vi "数据查询_仪器日志.vi"() -> ()   [LabVIEW 2016]
uses:
  <vilib>/Utility/miscctls.llb/LVRowAndColumnUnsignedTypeDef.ctl
  <vilib>/Utility/miscctls.llb/LVPointTypeDef.ctl
  <userlib>/_OpenG.lib/array/array.llb/Sort 2D Array (String)__ogtk.vi
panel:
  in  "序列号":string
  out "总共行数":i32
  in  "显示行数":i32=15
  in  "下拉列表":string(xcontrol)
  in  "导出":bool
  in  "查询":bool
  out "数据表":string[][](table)
  in  "结束日期":string="2050/01/01"
  in  "起始日期":string="2010/01/01"
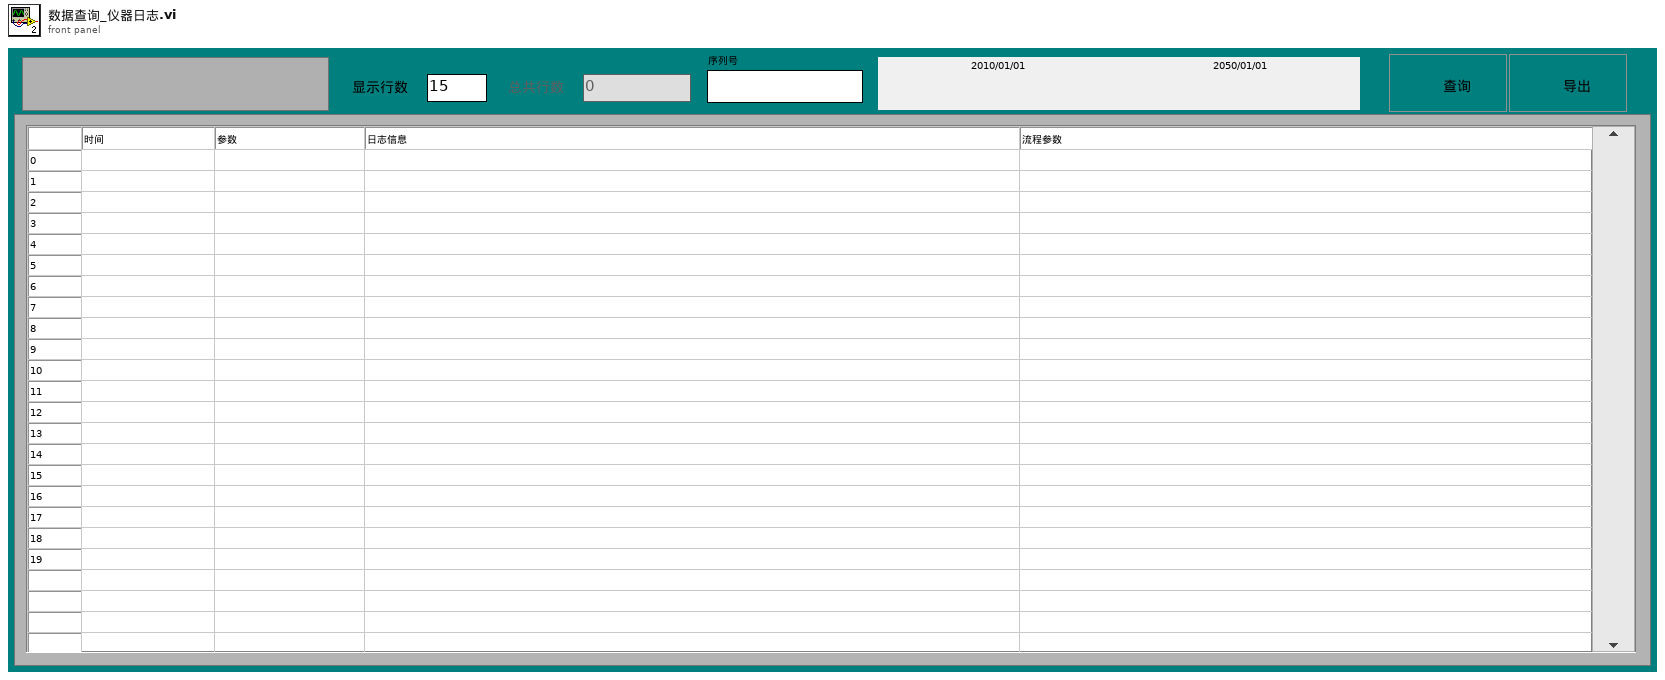
[diagram p1: front panel]
types:
  T1 = enum8{"Enabled", "Disabled", "Disabled and Grayed Out"}
  T2 = typedef "LVRowAndColumnUnsignedTypeDef.ctl" = cluster{"Row":u32, "Column":u32}
  T3 = typedef "LVPointTypeDef.ctl" = cluster{"Horizontal":i16, "Vertical":i16}
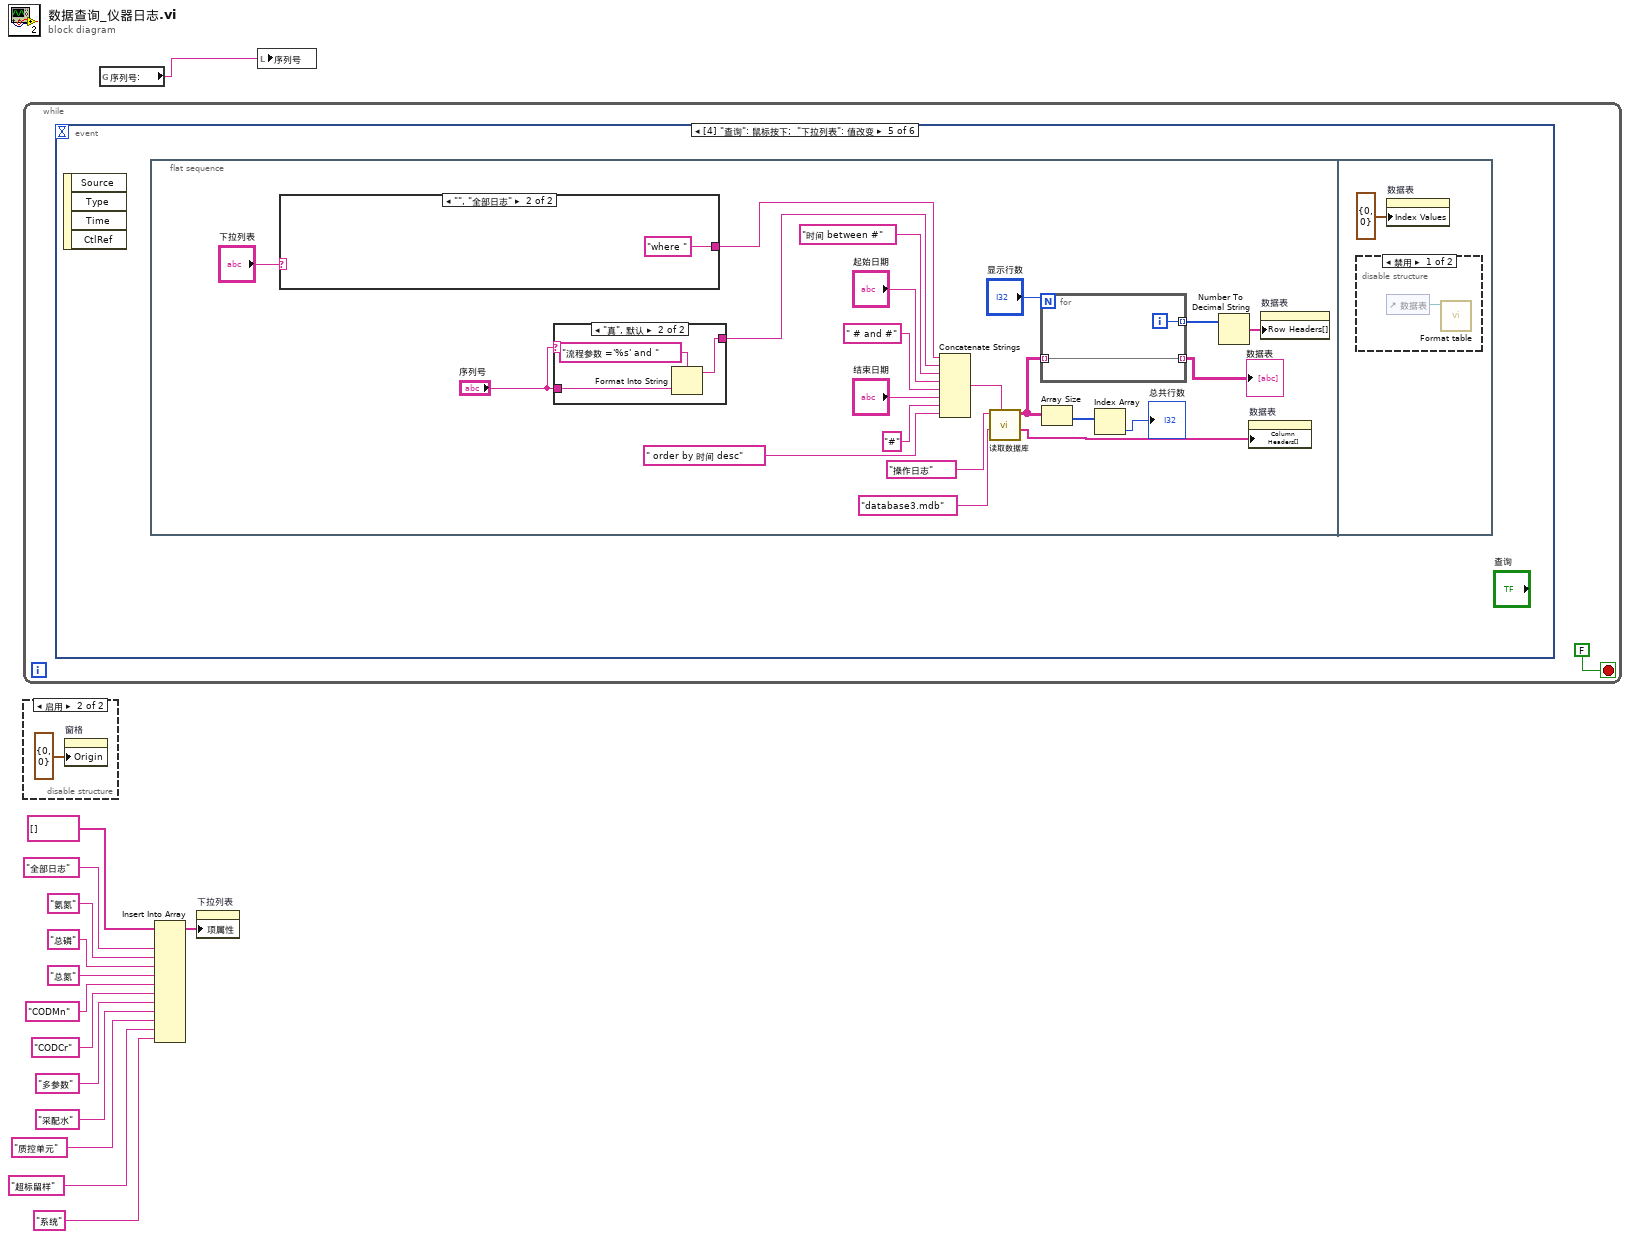
[diagram p0: block diagram]
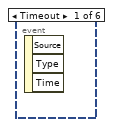
[diagram p2: hidden frame]
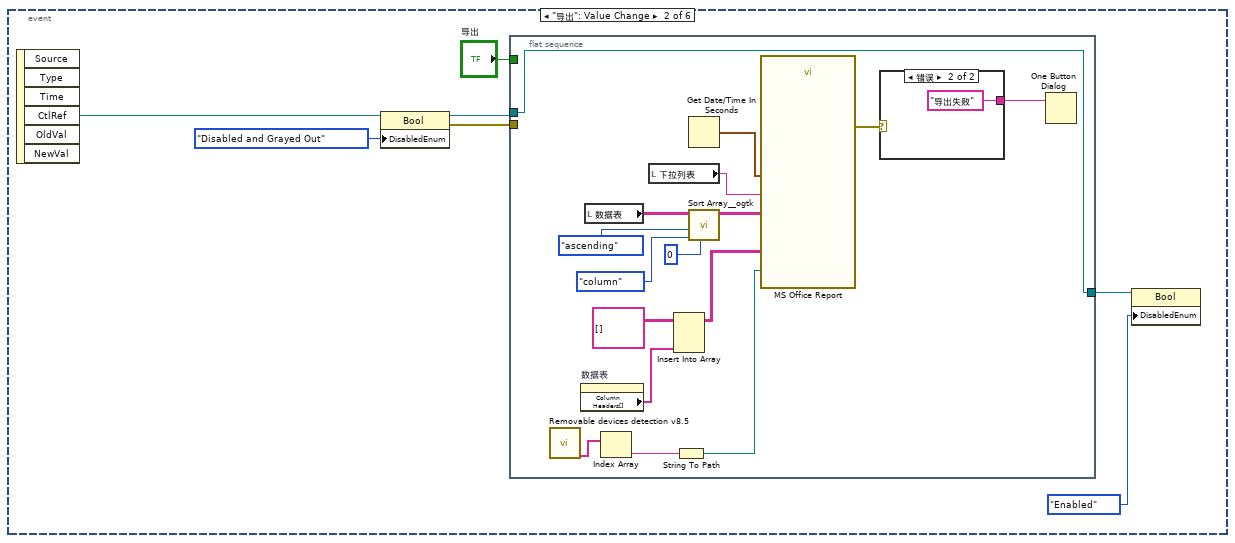
[diagram p3: hidden frame]
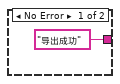
[diagram p4: hidden frame]
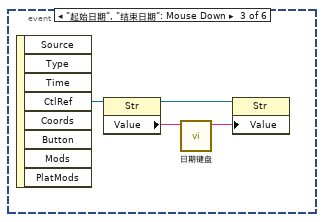
[diagram p5: hidden frame]
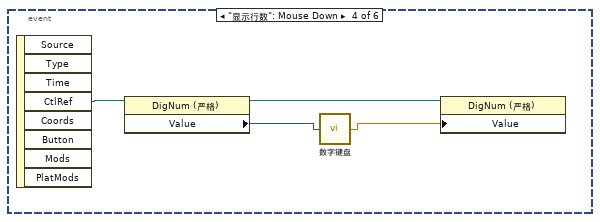
[diagram p6: hidden frame]
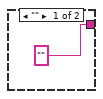
[diagram p7: hidden frame]
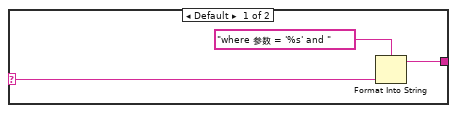
[diagram p8: hidden frame]
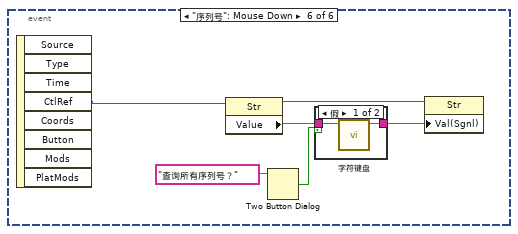
[diagram p10: hidden frame]
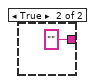
[diagram p11: hidden frame]
diagram:
  n1 = while {
    stop <- FALSE stop-if-true
    n2 = event shown="[4] \"查询\": 鼠标按下;  \"下拉列表\": 值改变" {
      selector: _ -> [_ _ _ _ _ _]
      dyn-events: _ -> [_ _ _ _ _ _]
      timeout: _ -> [_ _ _ _ _ _]
      event Timeout {
        n3 = event-data() -> ()  [unwired: 1 in, 3 out]
      }
      event "导出": Value Change {
        n4 = event-data() -> ("CtlRef"=w16:refnum<vi>)  [unwired: 1 in, 5 out]
        n5 = property class="Bool"(reference=w16, "DisabledEnum"=T1."Disabled and Grayed Out" ("禁用")) -> (reference out=w20:refnum<vi>, error out=w21:errorcluster)  [unwired: 1 in]
        n6 = flat-sequence {
          tunnel: w21 -> [_]
          tunnel: [w31] -> w19
          tunnel: w20 -> [w31]
          tunnel: "导出" -> [_]
          frame #0 {
            n7 = call "Removable devices detection v8.5.vi"() -> ("Removable"=w28:string[])  [unwired: 4 out]
            n8 = property on="数据表" class="Tbl (严格)"() -> ("Column Headers[]"=w23:string[])  [unwired: 2 in, 2 out]
            n9 = local read "数据表"() -> (w37:string[][])
            n10 = Index Array(array=w28) -> (element=w27:string)  [unwired: 1 in]
            n11 = local read "下拉列表"() -> (w32:string)
            n12 = Insert Into Array(array=string[][] [], new element=w23) -> (w24:string[][])  [unwired: 2 in]
            n13 = String To Path(string=w27) -> (path=w26:path)
            n14 = Get Date/Time In Seconds() -> (seconds since 1Jan1904=w38:timestamp)
            n15 = call-poly <userlib>:"Sort Array__ogtk.vi"("Column/Row to Sort By"=u32 0, "Sort By in"=enum16{"row", "column"}."column", "Order"=enum16{"ascending", "descending"}."ascending", "Array in"=w37) -> ("Sorted Array out"=w36:string[][])  [unwired: 4 in, 3 out]
            n16 = call "MS Office Report"("Path to Save Report"=w26, "导出日期"=w38, "监测参数"=w32, "数据输入"=w36, "字段定义"=w24) -> ("error out"=w30:errorcluster)  [unwired: 21 in, 1 out]
            n17 = case shown="错误" w30 {
              tunnel: ["导出成功" ("消息") "导出失败" ("消息")] -> w29
              frame No Error {
              }
              frame Error {
              }
            }
            n18 = One Button Dialog(message=w29) -> ()  [unwired: 1 in, 1 out]
          }
        }
        n19 = property class="Bool"(reference=w19, "DisabledEnum"=T1."Enabled" ("禁用")) -> ()  [unwired: 1 in, 2 out]
      }
      event "起始日期", "结束日期": Mouse Down {
        n20 = event-data() -> ("CtlRef"=w44:refnum<vi>)  [unwired: 1 in, 7 out]
        n21 = property class="Str"(reference=w44) -> (reference out=w42:refnum<vi>, "Value"=w43:string)  [unwired: 1 in, 1 out]
        n22 = call "日期键盘.vi"("原值"=w43) -> ("x+y"=w41:string)  [unwired: 10 in]
        n23 = property class="Str"(reference=w42, "Value"=w41) -> ()  [unwired: 1 in, 2 out]
      }
      event "显示行数": Mouse Down {
        n24 = event-data() -> ("CtlRef"=w48:refnum<vi>)  [unwired: 1 in, 7 out]
        n25 = property class="DigNum (严格)"(reference=w48) -> (reference out=w47:refnum<vi>, "Value"=w46:i32)  [unwired: 1 in, 1 out]
        n26 = call "数字键盘.vi"("OldNumber"=w46) -> ("NewNumber"=w45:sgl)
        n27 = property class="DigNum (严格)"(reference=w47, "Value"=w45) -> ()  [unwired: 1 in, 2 out]
      }
      event "查询": Mouse Down; "下拉列表": Value Change {
        n28 = event-data() -> ()  [unwired: 1 in, 4 out]
        n29 = flat-sequence {
          frame #0 {
            n30 = case shown="\"\", \"全部日志\"" "下拉列表" {
              selector: "下拉列表" -> [w74 _]
              tunnel: [w76 "where " ("condition")] -> w49
              frame Default {
                n31 = Format Into String(format string="where 参数 = '%s' and " ("condition"), w74) -> (resulting string=w76:string)  [unwired: 2 in, 1 out]
              }
              frame "", "全部日志" {
              }
            }
            n32 = case shown="\"真\", 默认" "序列号" {
              tunnel: "序列号" -> [_ w72]
              tunnel: ["" ("condition") w71] -> w51
              frame "" {
              }
              frame "真", Default {
                n33 = Format Into String(format string="流程参数 ='%s' and " ("condition"), w72) -> (resulting string=w71:string)  [unwired: 2 in, 1 out]
              }
            }
            n34 = Concatenate Strings(w49, w51, "时间 between #" ("condition"), "起始日期", " # and #" ("condition"), "结束日期", "#" ("condition"), " order by 时间 desc" ("字符串")) -> (w68:string)
            n35 = call "读取数据库.vi"("condition"=w68, "database"="database3.mdb", "组合框"="操作日志") -> ("columns"=w64:string[], "表格"=w55:string[][])  [unwired: 5 in, 2 out]
            n36 = for {
              N: "显示行数" -> [_]
              tunnel: w55 -> [w78] mode=indexing
              tunnel: [w79] -> w61 mode=indexing
              tunnel: [w78] -> w57 mode=indexing
              i -> [w79]
            }
            "数据表" <- w57
            n37 = Array Size(array=w55) -> (size(s)=w54:i32[])
            n38 = Index Array(array=w54) -> (element=→"总共行数":i32)  [unwired: 1 in]
            n39 = Number To Decimal String(number=w61) -> (decimal integer string=w60:string[])  [unwired: 1 in]
            n40 = property on="数据表" class="Tbl (严格)"("Column Headers[]"=w64) -> ()  [unwired: 2 in, 2 out]
            n41 = property on="数据表" class="Tbl (严格)"("Row Headers[]"=w60) -> ()  [unwired: 2 in, 2 out]
          }
          frame #1 {
            n42 = disable-structure shown="禁用" {
              frame Disabled {
                n43 = control-ref of="数据表"() -> (w81:refnum<vi>)
                n44 = call "Format table.vi"("Table输入"=w81) -> ()  [unwired: 11 in]
              }
              frame Enabled {
              }
            }
            n45 = property on="数据表" class="Tbl (严格)"("Index Values"=T2 {"Row"=0, "Column"=0} ("索引值")) -> ()  [unwired: 2 in, 2 out]
          }
        }
      }
      event "序列号": Mouse Down {
        n46 = event-data() -> ("CtlRef"=w82:refnum<vi>)  [unwired: 1 in, 7 out]
        n47 = property class="Str"(reference=w82) -> (reference out=w86:refnum<vi>, "Value"=w87:string)  [unwired: 1 in, 1 out]
        n48 = Two Button Dialog(message="查询所有序列号？" ("消息")) -> (T button?=w83:bool)  [unwired: 2 in]
        n49 = case shown="假" w83 {
          tunnel: w87 -> [w89 _]
          tunnel: [w88 "" ("x+y")] -> w85
          frame False {
            n50 = call "字符键盘.vi"("原值"=w89) -> ("x+y"=w88:string)  [unwired: 10 in]
          }
          frame True {
          }
        }
        n51 = property class="Str"(reference=w86, "Val(Sgnl)"=w85) -> ()  [unwired: 1 in, 2 out]
      }
    }
  }
  n52 = disable-structure shown="启用" {
    frame Disabled {
    }
    frame Enabled {
      n53 = property on="窗格" class="Pane"("Origin"=T3 {"Horizontal"=0, "Vertical"=0} ("原点")) -> ()  [unwired: 2 in, 2 out]
    }
  }
  n54 = global read "COD内部交互全局.vi" "序列号:"() -> (w1:string)
  n55 = Insert Into Array(array=string[] [], new element #1="全部日志" ("新元素/子数组"), new element #2="氨氮" ("新元素/子数组"), new element #3="总磷" ("新元素/子数组"), new element #4="总氮" ("新元素/子数组"), new element #5="CODMn" ("新元素/子数组"), new element #6="CODCr" ("新元素/子数组"), new element #7="多参数" ("新元素/子数组"), new element #8="采配水" ("新元素/子数组"), new element #9="质控单元" ("新元素/子数组"), new element #10="超标留样" ("新元素/子数组"), new element #11="系统" ("新元素/子数组")) -> (w5:string[])  [unwired: 1 in]
  n56 = property on="下拉列表" class="下拉列表 (严格)"("项属性"=w5) -> ()  [unwired: 2 in, 2 out]
  n57 = local write "序列号"(w1) -> ()
